vi "newMarkerSkill.vi"(7 "firstCall":bool, 8 "error in (no error)":errorcluster, 9 "Robot":refnum<class "Robot.lvclass">, 10 "Game":refnum<class "Game.lvclass">, 11 "MarkerSkill in":refnum<class "MarkerSkill.lvclass">) -> (0 "error out":errorcluster, 1 "numberOfPossible\nEnemiesToMark":i32, 2 "Robot out":refnum<class "Robot.lvclass">, 3 "MarkerSkill out":refnum<class "MarkerSkill.lvclass">)   [LabVIEW 2023, in "MarkerSkill.lvclass"]
uses:
  MarkerSkill.lvclass
  Robot_class/Robot.lvclass
  Game_class/Game.lvclass
  Referee_class/command_interpreted.ctl
  dangerEnemy.ctl
  Game_class/Game.lvclass/Game.ctl
  Team_class/Team.lvclass/Team.ctl
  Object_class/Object.lvclass/Object.ctl
  Parameters_class/Parameters.lvclass/Parameters.ctl
  Referee_class/Referee.lvclass/Referee.ctl
  Field_class/Field.lvclass/Field.ctl
  Robot_class/Robot.lvclass/Robot.ctl
  440f4cb0-977a-49d7-a6a6-20607285011f.vi
  <vilib>/Analysis/baseanly.llb/Unit Vector (DBL).vi
  Game_class/Read BallRef.vi
  Game_class/Read Referee.vi
  Game_class/Read Parameters.lvclass.vi
  Parameters_class/Read DistanceStop.vi
  Referee_class/Read command_interpreted.vi
  Object_class/Read x.vi
  Object_class/Read y.vi
  Game_class/Read OffensiveTeam.vi
  Game_class/Read EnemyRef.vi
  Game_class/Read FieldRef.vi
  Game_class/Read NewParameters.vi
  Parameters_class/Read Type of Marker.vi
  Field_class/Read ourGoalPosition.vi
  Object_class/Read position(x,y).vi
  Team_class/Read RobotRef.vi
  Robot_class/Read id.vi
  Robot_class/Write dest_x.vi
  Robot_class/Write dest_y.vi
  Robot_class/Write dest_orientation.vi
  Ball_class/Ball.lvclass
  C:/Users/ebert/Documents/codes/SSL/repo/SSL_AI/Object_class/Object.lvclass
  Enemy_class/Enemy.lvclass
  C:/Users/ebert/Documents/codes/SSL/repo/SSL_AI/Team_class/Team.lvclass
  Ally_class/Ally.lvclass
  Field_class/Field.lvclass
  Parameters_class/Parameters.lvclass
  Referee_class/Referee.lvclass
  <vilib>/Comparison/Less/Less Functor/Less Functor.lvclass
  MarkerSkill.lvclass/MarkerSkill.ctl
  Utilities_class/Utilities.lvclass
  <vilib>/Analysis/NI_AALBase.lvlib
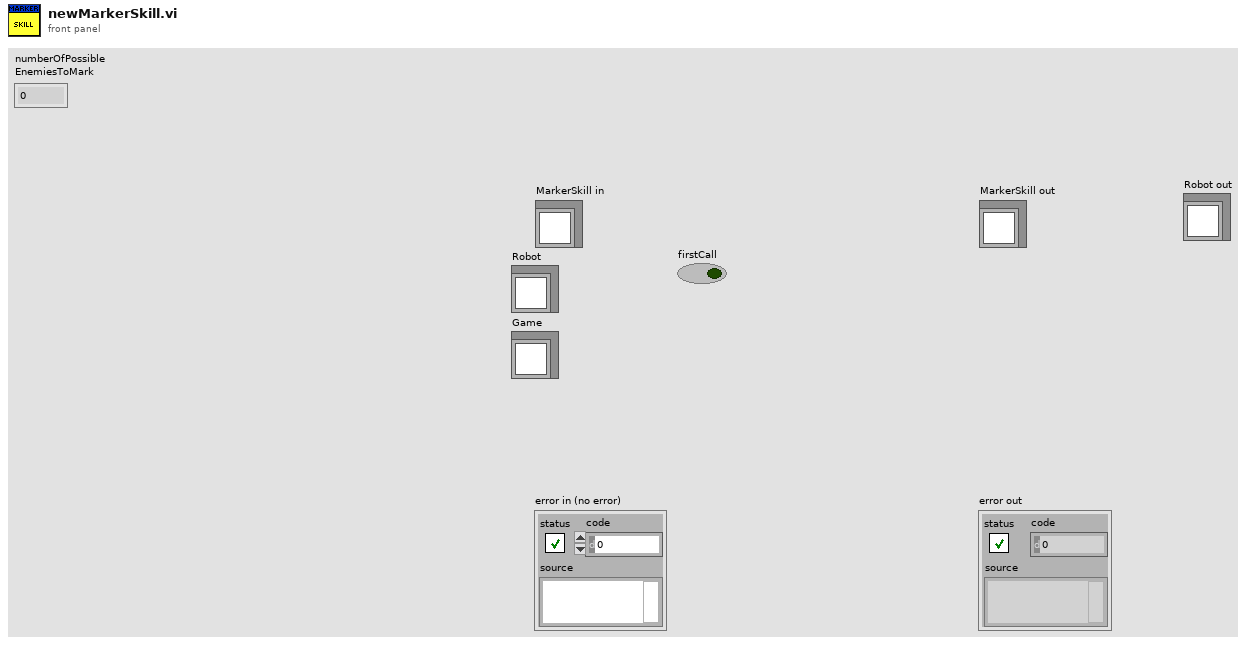
[diagram p1: front panel]
types:
  T1 = typedef "dangerEnemy.ctl" = cluster{"dangerFactor":dbl, "allyRobotId":i32, "enemyRobotId":i32}
  T2 = typedef "command_interpreted.ctl" = enum16{"Goal Ally", "Goal Enemy", "Ball Placement Enemy", "Ball Placement Ally", "Normal Half Time", "Extra Time  Break", "Extra Half Time", "None", "Post Game", "PKA Normal Start", "Prepare Kickoff Ally", "PKE Normal Start", "Prepare Kickoff Enemy", "Force Start", "Halt", "Timeout", "Prepare Penalty Ally", "Prepare Penalty Enemy", "PPA NormalStart", "PPE Normal Start", "Indirect Free Ally", "Direct Free Enemy", "Direct Free Ally", "Indirect Free Enemy", "Stop"}
  T3 = typedef "NewParameters.ctl" = cluster{"PenaltyDistance":dbl, "DistanceAttackerToBackBall":dbl, "Division":enum16{"Div B", "Div A"}, "DistanceToAvoidyEnemyRobot":dbl, "BallPlacementDistance":dbl, "DisatanceBehindBallToStealBall":dbl, "MaxDistanceToPositionKickoff":dbl, "BlockEnemyTarget":bool, "MaxStopVAng":dbl, "DistanceMarkerToEnemy":dbl, "IgnoreDribblerContact":bool, "DistanceToBeginEnemyPosession":dbl, "GoToBallWhenEnemyNotMoving":bool, "EnemyDistanceToReduceVelocity":dbl, "TurnOnEnemyDistanceToReduceVelocity":bool, "EnemyDistanceToShootOutBall":dbl, "DefenseKickBall":bool, "MoreKickToGoal? (0-0.3)":dbl, "ChipKickInEnemyField":bool, "ShootOutRobotId":dbl, "FieldLenghtDenominatorInShootOut":dbl, "AdjustPositionInBallPlacement":bool, "PowerGodPass":dbl, "VelocityAbortEnemyPos":dbl, "MaxDistToBeginPass":dbl, "MinDistToBeginPass":dbl, "VelocityInDirects":dbl, "BadDribblerIDs":i32[], "NewKickToDistanceAroundBall":dbl, "PowerAvoidColisionMarker":dbl, "DistanceToAvoidColisionMarker":dbl, "AvoidBallKick":dbl, "DistanceTryKick":dbl, "SuicideKickDIstance":dbl, "FirstKickAtck":bool, "AdjustFirstKickDistance":dbl, "FirstKickDefense":bool, "AvoidAimLessKick":dbl, "DistanceToAvoidyEnemyShootRobot ":dbl, "NumberOfMarkers":dbl, "PotField":bool, "PIDLateral":bool, "MinDistanceFirstKickX":dbl, "MinDistanceFirstKickY":dbl, "FractionOfDistToTouchGround\nAfterChipKick":dbl, "FractionOfKickxWhen\nComposedWithKickz":dbl, "Style":T4, "MoveInTurnState":bool, "DistFromEnemyToConsider\nMoveInTurnState":dbl, "CascadePID":bool, "TurnAroundParameters":cluster{"Radius":dbl, "Multiplier":dbl, "ChordAngle":dbl}, "SafeDriveVel":dbl, "DistanceToGoToBackBall":dbl, "minDistanceToNotFinishEnemyPossession":dbl, "Probability to kick direct penalty (0 - 1)":dbl}
  T4 = typedef "Style.ctl" = enum16{"Insanity", "Offensive", "Defensive"}
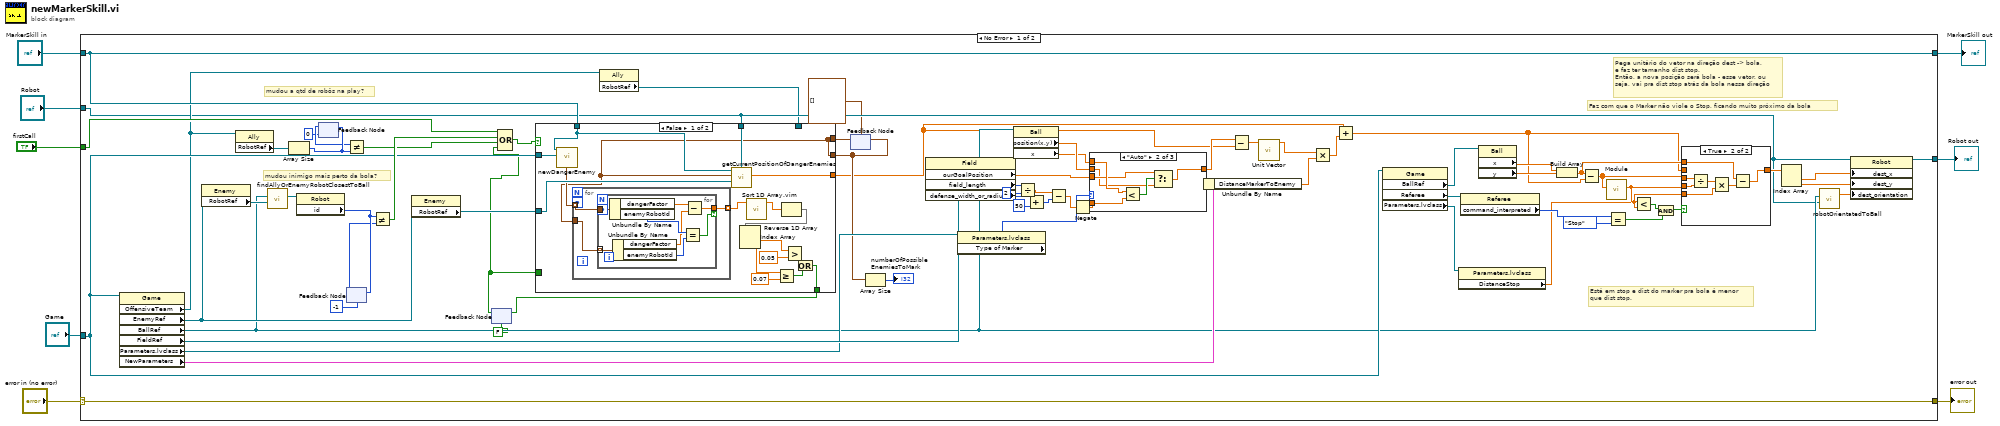
[diagram p0: block diagram]
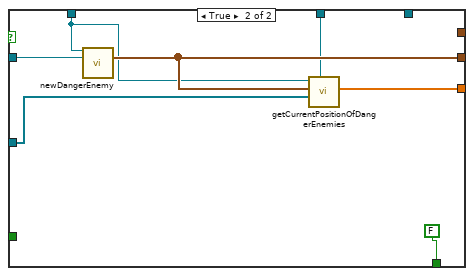
[diagram p2: hidden frame]
diagram:
  n1 = case shown="No Error" "error in (no error)" {
    selector: "error in (no error)" -> [w78 w131]
    tunnel: [w78 w131] -> w7
    tunnel: [w51 w130] -> w5
    tunnel: "MarkerSkill in" -> [w51 w130]
    tunnel: "Game" -> [w47 _]
    tunnel: "Robot" -> [w25 _]
    tunnel: "firstCall" -> [w60 _]
    tunnel: [w39 _] -> w1
    frame No Error {
      # "mudou inimigo mais perto da bola?"
      # "mudou a qtd de robôs na play?"
      # "Pega unitário do vetor na direção dest -> bola,\ne faz ter tamanho dist stop.\nEntão, a nova posição será bola - esse vetor, ou\nseja, vai pra dist stop atrás da bola nessa direção"
      # "Está em stop e dist do marker pra bola é menor\nque dist stop."
      # "Faz com que o Marker não viole o Stop, ficando muito próximo da bola"
      n2 = property class="Game"(reference=w47) -> ("OffensiveTeam"=w31:refnum<class "Ally.lvclass">, "EnemyRef"=w58:refnum<class "Enemy.lvclass">, "BallRef"=w34:refnum<class "Ball.lvclass">, "FieldRef"=w67:refnum<class "Field.lvclass">, "Parameters.lvclass"=w59:refnum<class "Parameters.lvclass">, "NewParameters"=w43:T3)  [unwired: 1 in, 2 out]
      n3 = property class="Enemy"(reference=w58) -> ("RobotRef"=w57:refnum<class "Robot.lvclass">[])  [unwired: 1 in, 2 out]
      n4 = property class="Ally"(reference=w31) -> ("RobotRef"=w30:refnum<class "Robot.lvclass">[])  [unwired: 1 in, 2 out]
      n5 = call "findAllyOrEnemyRobotClosestToBall.vi"("Ally/Enemy Robots"=w57, "Ball"=w34) -> ("Robot"=w56:refnum<class "Robot.lvclass">)  [unwired: 5 in, 4 out]
      n6 = Array Size(array=w30) -> (size(s)=w29:i32)
      n7 = property class="Robot"(reference=w56) -> ("id"=w55:i32)  [unwired: 1 in, 2 out]
      n8 = feedback-in #1(w29) -> ()
      n9 = feedback #1(0) -> (w28:i32)
      n10 = feedback #2(-1 ("id")) -> (w54:i32)
      n11 = feedback-in #2(w55) -> ()
      n12 = Not Equal?(x=w28, y=w29) -> (x != y?=w27:bool)
      n13 = Not Equal?(x=w55, y=w54) -> (x != y?=w52:bool)
      n14 = property class="Enemy"(reference=w58) -> ("RobotRef"=w61:refnum<class "Robot.lvclass">[])  [unwired: 1 in, 2 out]
      n15 = feedback #3(FALSE) -> (w17:bool)
      n16 = Compound Arithmetic op=OR(w60, w52, w27, w17) -> (w19:bool)
      n17 = property class="Ally"(reference=w31) -> ("RobotRef"=w24:refnum<class "Robot.lvclass">[])  [unwired: 1 in, 2 out]
      n18 = feedback #4(T1[] [] ("dangerEnemies")) -> (w62:T1[])
      n19 = case shown="False" w19 {
        tunnel: [w89 w112] -> w33
        tunnel: w47 -> [w92 w113]
        tunnel: w51 -> [w91 w110]
        tunnel: w62 -> [w89 _]
        tunnel: w61 -> [w95 w111]
        tunnel: w25 -> [w94 w108]
        tunnel: w24 -> [_ _]
        tunnel: [w93 w109] -> w23
        tunnel: [w79 FALSE] -> w20
        tunnel: w17 -> [_ _]
        frame False {
          n20 = call "newDangerEnemy.vi"("MarkerSkill in"=w91, "Game"=w92) -> ("dangerEnemies"=w90:T1[])  [unwired: 10 in, 3 out]
          n21 = for {
            tunnel: w90 -> [w98] mode=indexing
            tunnel: w89 -> [w96]
            tunnel: [w97] -> w88 mode=indexing
            workers-P: _ -> [_]
            n22 = for {
              tunnel: w98 -> [w106]
              tunnel: [w101] -> w97 if=w99
              tunnel: w96 -> [w100] mode=indexing
              workers-P: _ -> [_]
              n23 = Unbundle By Name(w106) -> ("dangerFactor"=w103:dbl, "enemyRobotId"=w104:i32)
              n24 = Unbundle By Name(w100) -> ("dangerFactor"=w102:dbl, "enemyRobotId"=w105:i32)
              n25 = Equal?(x=w104, y=w105) -> (x = y?=w99:bool)
              n26 = Subtract(x=w103, y=w102) -> (x-y=w101:dbl)
            }
          }
          n27 = call "getCurrentPositionOfDangerEnemies.vi"("Robot"=w94, "RobotRef"=w95, "dangerEnemies"=w89, "MarkerSkill in"=w91) -> ("positionToMark"=w93:dbl[])  [unwired: 5 in, 2 out]
          n28 = call "Sort 1D Array.vim"("unsorted array"=w88) -> ("sorted array"=w87:dbl[])  [unwired: 10 in]
          n29 = Reverse 1D Array(array=w87) -> (reversed array=w86:dbl[])
          n30 = Index Array(array=w86) -> (element #1=w84:dbl, element #2=w83:dbl)  [unwired: 2 in]
          n31 = Greater Or Equal?(x=w83, y=0.07) -> (x >= y?=w80:bool)
          n32 = Greater?(x=w84, y=0.05) -> (0:w81:bool)
          n33 = Or(x=w81, y=w80) -> (x .or. y?=w79:bool)
        }
        frame True {
          n34 = call "newDangerEnemy.vi"("MarkerSkill in"=w110, "Game"=w113) -> ("dangerEnemies"=w112:T1[])  [unwired: 10 in, 3 out]
          n35 = call "getCurrentPositionOfDangerEnemies.vi"("Robot"=w108, "RobotRef"=w111, "dangerEnemies"=w112, "MarkerSkill in"=w110) -> ("positionToMark"=w109:dbl[])  [unwired: 5 in, 2 out]
        }
      }
      n36 = feedback-in #3(w20) -> ()
      n37 = feedback-in #4(w33) -> ()
      n38 = Array Size(array=w33) -> (size(s)=→"numberOfPossible\nEnemiesToMark":i32)
      n39 = property class="Field"(reference=w67) -> ("ourGoalPosition"=w50:dbl[], "field_length"=w16:i32, "defense_width_or_radius"=w13:i32)  [unwired: 1 in, 2 out]
      n40 = property class="Parameters.lvclass"(reference=w59) -> ("Type of Marker"=w49:enum16{"Auto", "BlockEnemyPass", "BlockOurGoal"})  [unwired: 1 in, 2 out]
      n41 = property class="Ball"(reference=w34) -> ("position(x,y)"=w48:dbl[], "x"=w22:dbl)  [unwired: 1 in, 2 out]
      n42 = Divide(x=w16, y=2) -> (x/y=w14:dbl)
      n43 = Add(x=w13, y=50) -> (x+y=w11:i32)
      n44 = Subtract(x=w14, y=w11) -> (x-y=w10:dbl)
      n45 = Negate(x=w10) -> (-x=w9:dbl)
      n46 = case shown="\"Auto\"" w49 {
        tunnel: [w114 w120 w121] -> w45
        tunnel: w50 -> [_ w116 w121]
        tunnel: w48 -> [w114 w115 _]
        tunnel: w22 -> [_ w119 _]
        tunnel: w9 -> [_ w118 _]
        frame "BlockEnemyPass", Default {
        }
        frame "Auto" {
          n47 = Less?(x=w119, y=w118) -> (x < y?=w117:bool)
          n48 = Select(t=w116, s=w117, f=w115) -> (s? t:f=w120:dbl[])
        }
        frame "BlockOurGoal" {
        }
      }
      n49 = Unbundle By Name(w43) -> ("DistanceMarkerToEnemy"=w41:dbl)
      n50 = Subtract(x=w45, y=w23) -> (x-y=w44:dbl[])
      n51 = call-poly <vilib>:"Unit Vector.vi"("Input Vector"=w44) -> ("Unit Vector"=w42:dbl[])  [unwired: 8 in, 2 out]
      n52 = Multiply(x=w42, y=w41) -> (x*y=w40:dbl[])
      n53 = Add(x=w23, y=w40) -> (x+y=w46:dbl[])
      n54 = property class="Game"(reference=w47) -> ("BallRef"=w73:refnum<class "Ball.lvclass">, "Referee"=w70:refnum<class "Referee.lvclass">, "Parameters.lvclass"=w64:refnum<class "Parameters.lvclass">)  [unwired: 1 in, 2 out]
      n55 = property class="Parameters.lvclass"(reference=w64) -> ("DistanceStop"=w63:dbl)  [unwired: 1 in, 2 out]
      n56 = property class="Referee"(reference=w70) -> ("command_interpreted"=w69:T2)  [unwired: 1 in, 2 out]
      n57 = property class="Ball"(reference=w73) -> ("x"=w72:dbl, "y"=w71:dbl)  [unwired: 1 in, 2 out]
      n58 = Build Array(w72, w71) -> (w74:dbl[])
      n59 = Subtract(x=w74, y=w46) -> (x-y=w66:dbl[])
      n60 = call "Module.vi"("2D vector"=w66) -> ("Modulo"=w65:dbl)  [unwired: 8 in, 2 out]
      n61 = Equal?(x=w69, y=command_interpreted."Stop") -> (x = y?=w76:bool)
      n62 = Less?(x=w65, y=w63) -> (x < y?=w77:bool)
      n63 = And(x=w77, y=w76) -> (x .and. y?=w75:bool)
      n64 = case shown="True" w75 {
        tunnel: [w122 w124] -> w38
        tunnel: w46 -> [w122 _]
        tunnel: w65 -> [_ w129]
        tunnel: w63 -> [_ w127]
        tunnel: w74 -> [_ w126]
        tunnel: w66 -> [_ w123]
        frame False {
        }
        frame True {
          n65 = Divide(x=w123, y=w129) -> (x/y=w128:dbl[])
          n66 = Multiply(x=w128, y=w127) -> (x*y=w125:dbl[])
          n67 = Subtract(x=w126, y=w125) -> (x-y=w124:dbl[])
        }
      }
      n68 = Index Array(array=w38) -> (element #1=w37:dbl, element #2=w36:dbl)  [unwired: 2 in]
      n69 = call "robotOrientatedToBall.vi"("Robot"=w25, "BallRef"=w34) -> ("Orientation"=w35:dbl)  [unwired: 7 in, 2 out]
      n70 = property class="Robot"(reference=w25, "dest_x"=w37, "dest_y"=w36, "dest_orientation"=w35) -> (reference out=w39:refnum<class "Robot.lvclass">)  [unwired: 1 in, 1 out]
    }
    frame Error {
    }
  }
  "error out" <- w7
  "MarkerSkill out" <- w5
  "Robot out" <- w1
